vi "Check Until Not Busy.vi"(8 "error in":errorcluster, 11 "LCD in":refnum<class "Character LCD.lvclass">) -> (0 "error out":errorcluster, 3 "LCD out":refnum<class "Character LCD.lvclass">)   [LabVIEW 2015]
uses:
  <vilib>/EmbeddedDisplay/Hitachi HD44780/Host/Internal/LCD Class/Character LCD.lvclass
  <vilib>/EmbeddedDisplay/Hitachi HD44780/Host/HD44780 Host.lvlib
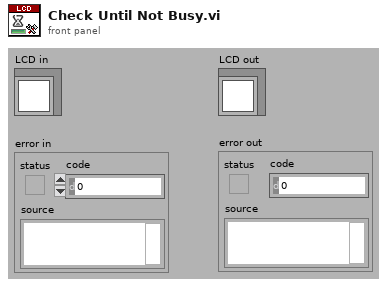
[diagram p1: front panel]
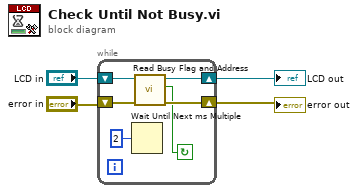
[diagram p0: block diagram]
diagram:
  n1 = while {
    shift-right: [w7] -> w1
    shift-left: "error in" -> [w8]
    shift-right: [w9] -> w2
    shift-left: "LCD in" -> [w10]
    stop <- w6 continue-if-true
    n2 = Wait Until Next ms Multiple(millisecond multiple=u32 2) -> ()  [unwired: 1 out]
    n3 = call <vilib>:"Read Busy Flag and Address.vi"("error in (no error)"=w8, "LCD in"=w10) -> ("error out"=w7:errorcluster, "busy flag"=w6:bool, "LCD out"=w9:refnum<class "Character LCD.lvclass">)  [unwired: 6 in, 1 out]
  }
  "LCD out" <- w2
  "error out" <- w1
